vi "读取状态.vi"(8 "error in (no error)":errorcluster caption="错误输入（无错误）", 11 "信号灯成员类.lvclass输入":refnum<class "信号灯成员类.lvclass">) -> (0 "error out":errorcluster caption="错误输出", 1 "状态":enum16{"绿灯亮", "黄灯亮", "红灯亮", "全部亮", "全部熄灭"}(ring), 3 "信号灯成员类.lvclass输出":refnum<class "信号灯成员类.lvclass">)   [LabVIEW 2017, in "信号灯成员类.lvclass"]
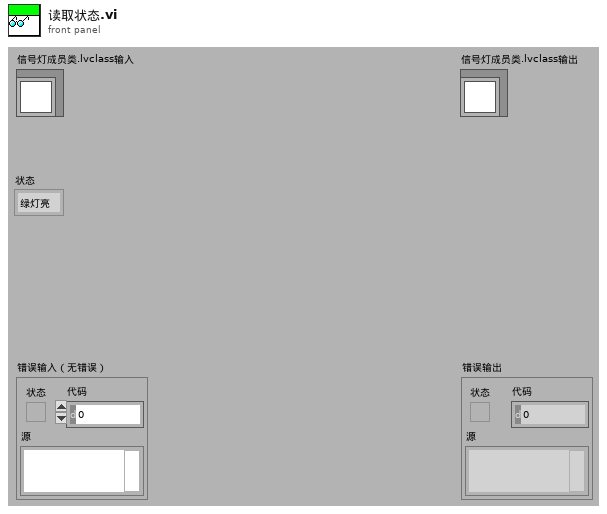
[diagram p1: front panel]
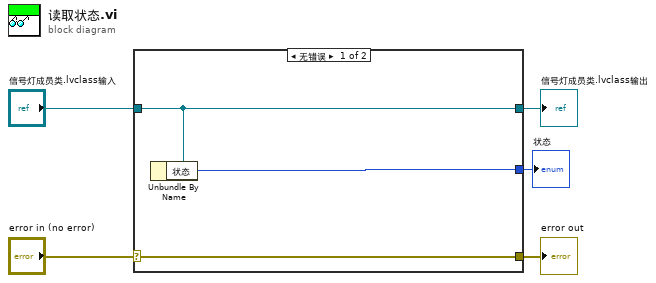
[diagram p0: block diagram]
diagram:
  n1 = case shown="无错误" "error in (no error)" {
    selector: "error in (no error)" -> [w8 w9]
    tunnel: [w8 w9] -> w4
    tunnel: [w7 w10] -> w2
    tunnel: "信号灯成员类.lvclass输入" -> [w7 w10]
    tunnel: [w6 _] -> w1
    frame No Error {
      n2 = Unbundle By Name(w7) -> ("状态"=w6:enum16{"绿灯亮", "黄灯亮", "红灯亮", "全部亮", "全部熄灭"})
    }
    frame Error {
    }
  }
  "error out" <- w4
  "信号灯成员类.lvclass输出" <- w2
  "状态" <- w1
